vi "test_number_selector.vi"(0 "1st tst in":dbl, 2 "2nd tst in":dbl, 3 "test mode":T1(ring)) -> (5 "1st tst out":dbl, 6 "2nd tst out":dbl)   [LabVIEW 2015]
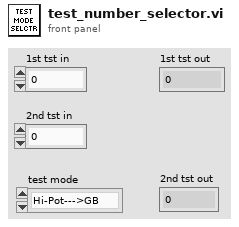
[diagram p1: front panel]
types:
  T1 = enum16{"Hi-Pot--->GB", "GB--->Hi-Pot", "Hi-Pot only", "GB only"}
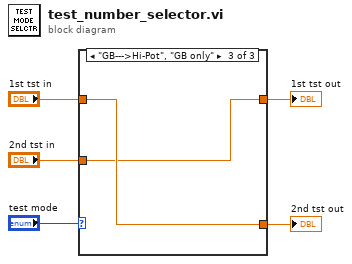
[diagram p0: block diagram]
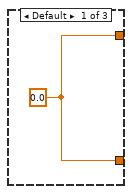
[diagram p2: hidden frame]
diagram:
  n1 = case shown="\"GB--->Hi-Pot\", \"GB only\"" "test mode" {
    tunnel: "1st tst in" -> [_ w8 w10]
    tunnel: "2nd tst in" -> [_ w7 w9]
    tunnel: [w6 w8 w9] -> w3
    tunnel: [w6 w7 w10] -> w2
    frame Default {
      w6 = 0.0
    }
    frame "Hi-Pot--->GB", "Hi-Pot only" {
    }
    frame "GB--->Hi-Pot", "GB only" {
    }
  }
  "1st tst out" <- w3
  "2nd tst out" <- w2
